vi "Find Message.vi"(8 "error in":errorcluster, 10 "message name":string, 11 "port in":T1 format="%.0x") -> (0 "error out":errorcluster, 2 "message refs":T1[](array[typedef]) format="%.0x", 3 "port out":T1 format="%.0x", 4 "found?":bool)   [LabVIEW 2020, in "Ballard MIL-STD-1553 Scripting.lvlib"]
doc: "Within the specified <b>port in</b>, searches for instances of <b>message name</b>. If a match is found, returns the matching <b>message refs</b>. If no match is found, the array of returned references is empty and <b>found?</b> equals False."
uses:
  Ballard MIL-STD-1553 Scripting.lvlib
  <vilib>/NI VeriStand/Custom Device API/Custom Device Item Ref.ctl
  <vilib>/NI VeriStand/Custom Device API/Custom Device API.lvlib
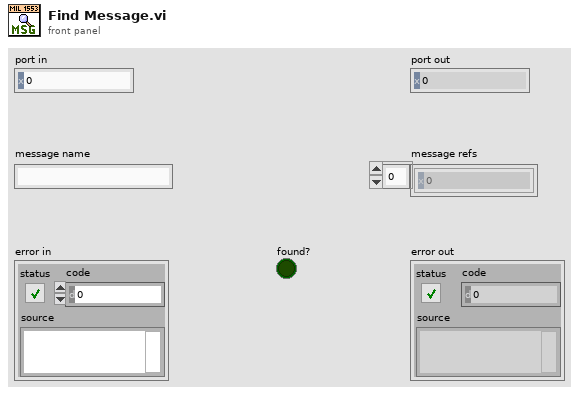
[diagram p1: front panel]
types:
  T1 = typedef "Custom Device API.lvlib/Custom Device Item Ref.ctl" = u64
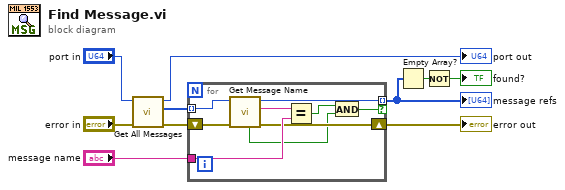
[diagram p0: block diagram]
diagram:
  n1 = call "Get All Messages.vi"("error in"="error in", "port in"="port in") -> ("error out"=w5:errorcluster, "messages"=w8:T1[], "port out"=→"port out":T1)  [unwired: 7 in]
  n2 = for {
    tunnel: w8 -> [w19] mode=indexing
    tunnel: "message name" -> [w18]
    tunnel: [w13] -> w3 mode=indexing if=w11
    shift-right: [w14] -> w4
    shift-left: w5 -> [w15]
    n3 = call "Get Message Name.vi"("error in"=w15, "message in"=w19) -> ("error out"=w14:errorcluster, "message name"=w17:string, "message out"=w13:T1, "found?"=w12:bool)  [unwired: 6 in]
    n4 = Equal?(x=w17, y=w18) -> (x = y?=w16:bool)
    n5 = And(x=w16, y=w12) -> (x .and. y?=w11:bool)
  }
  "error out" <- w4
  "message refs" <- w3
  n6 = Empty Array?(array=w3) -> (empty?=w1:bool)
  n7 = Not(x=w1) -> (.not. x?=→"found?":bool)
